vi "Checksum_2.vi"(1 "input array":u8[](array[numeric])) -> (0 "output array":u8[](array[numeric]))   [LabVIEW 2014]
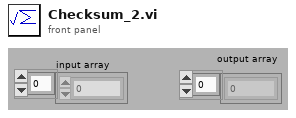
[diagram p1: front panel]
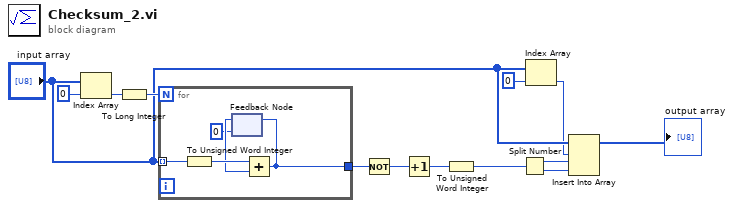
[diagram p0: block diagram]
diagram:
  n1 = Index Array(array="input array", index=0) -> (element=w13:u8)
  n2 = To Long Integer(number=w13) -> (32bit integer=w12:i32)
  n3 = for {
    N: w12 -> [_]
    tunnel: "input array" -> [w18] mode=indexing
    tunnel: [w15] -> w7
    n4 = To Unsigned Word Integer(number=w18) -> (unsigned 16bit integer=w17:u16)
    n5 = feedback #1(u16 0) -> (w16:u16)
    n6 = Add(x=w17, y=w16) -> (x+y=w15:u16)
    n7 = feedback-in #1(w15) -> ()
  }
  n8 = Not(x=w7) -> (.not. x?=w6:u16)
  n9 = Increment(x=w6) -> (x+1=w5:u16)
  n10 = To Unsigned Word Integer(number=w5) -> (unsigned 16bit integer=w4:u16)
  n11 = Split Number(x=w4) -> (hi(x)=w3:u8, lo(x)=w2:u8)
  n12 = Index Array(array="input array", index=0) -> (element=w8:u8)
  n13 = Insert Into Array(array="input array", index=w8, new element #1=w3, new element #2=w2) -> (→"output array":u8[])
